vi "dV(dRo).vi"(1 "stop":bool, 4 "dRo /dC":dbl, 6 "dRo %":dbl format="%#_3g", 8 "C подпитка":dbl, 9 "T1к-р C":dbl, 10 "N ГЦП":dbl, 11 "C крайно":dbl) -> (0 "dC г/кг":dbl format="%#_3g", 2 "L см":dbl format="%#_3f", 3 "V м3":dbl format="%#_3f")   [LabVIEW 2023]
panel:
  out "Дозирай на всеки 10 сек за:":dbl format="%#_2g"
  in  "∆L sm":dbl
  in  "F m3/h":dbl
  in  "dN/dt %/h":dbl
  in  "∆N %":dbl
  out "dRo % 2":dbl format="%#_3g"
  in  "dC г/кг 2":dbl format="%#_3g"
  in  "dRo /dC 2":dbl
  out "date/time string":string
  out "V 1к-р":dbl format="%#_3f"
  out "Enum":enum16{"Хов", "Бор"}(ring)
  in  "C начално":dbl
  out "x > y?":bool
  # "сек"
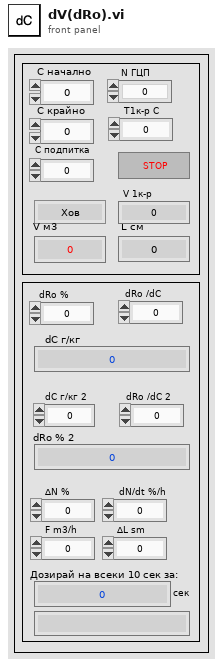
[diagram p1: front panel]
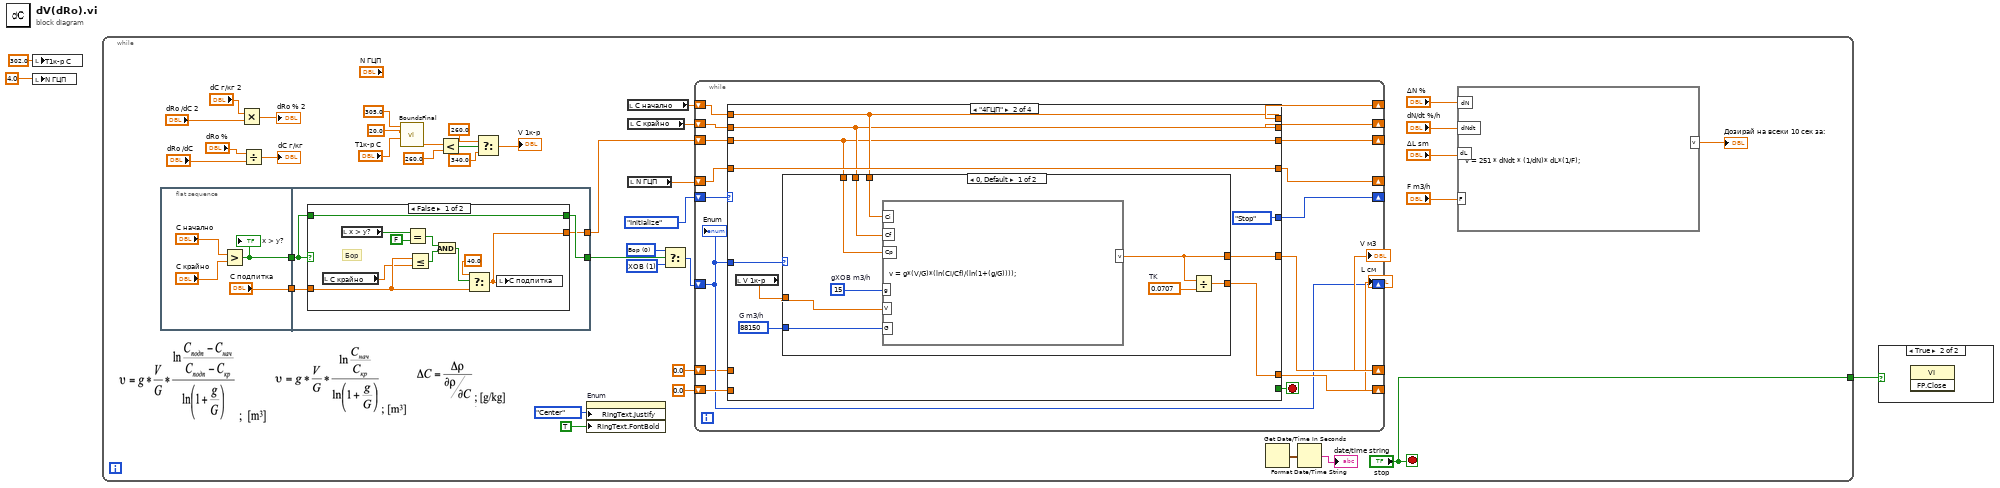
[diagram p0: block diagram]
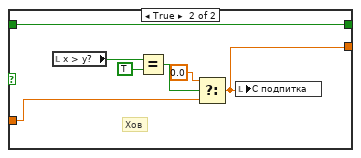
[diagram p3: hidden frame]
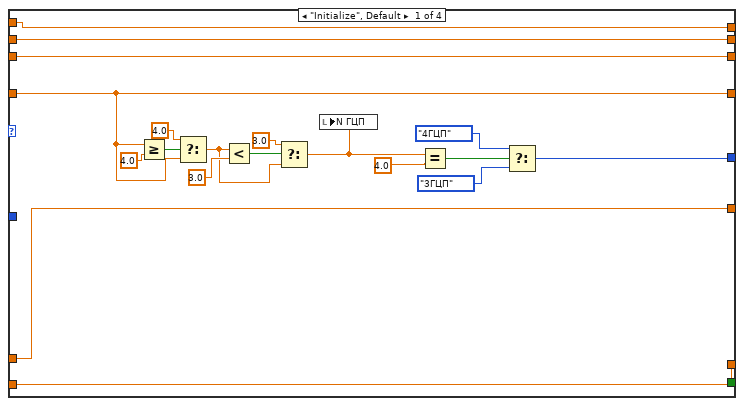
[diagram p4: hidden frame]
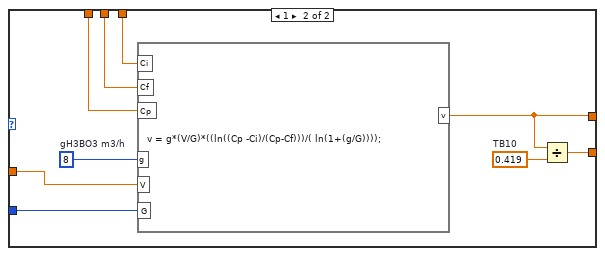
[diagram p5: hidden frame]
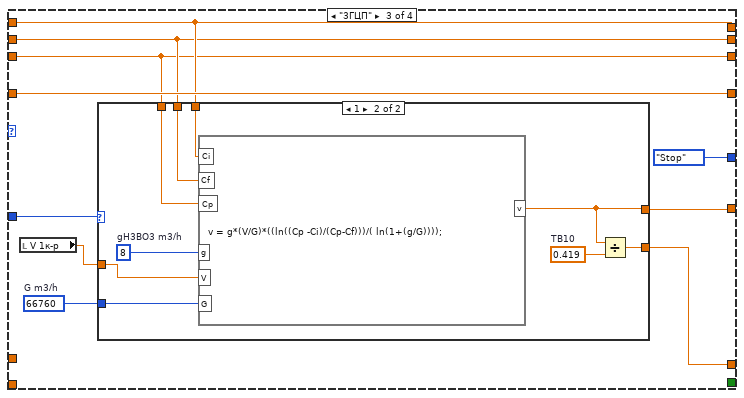
[diagram p6: hidden frame]
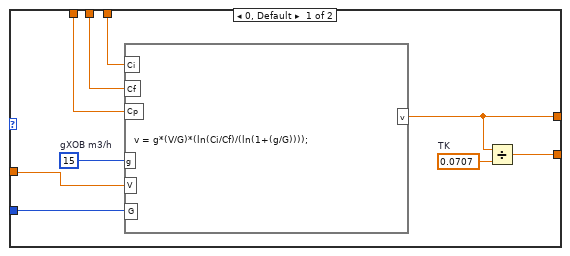
[diagram p7: hidden frame]
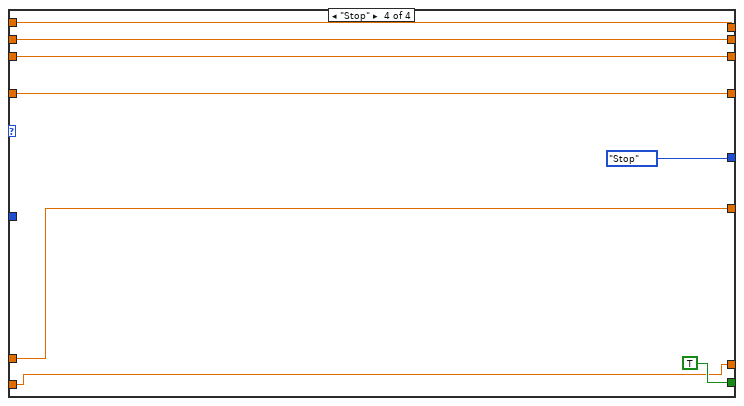
[diagram p8: hidden frame]
diagram:
  n1 = local write "T1к-р C"(302.0) -> ()
  n2 = local write "N ГЦП"(4.0) -> ()
  n3 = while {
    tunnel: ["stop"] -> w3
    stop <- "stop" stop-if-true
    w37 = u16 0 items=["Бор", "ХОВ"]
    w38 = u16 1 items=["Бор", "ХОВ"]
    n4 = flat-sequence {
      tunnel: [w47] -> w43
      tunnel: ["C подпитка"] -> w42
      tunnel: [w50] -> w33
      tunnel: w43 -> [w51]
      tunnel: [w49] -> w32
      tunnel: w42 -> [w48]
      frame #0 {
        n5 = Greater?(x="C начално", y="C крайно") -> (0:w47:bool)
        "x > y?" <- w47
      }
      frame #1 {
        n6 = case shown="False" w51 {
          tunnel: w51 -> [w55 w68]
          tunnel: [w55 w68] -> w50
          tunnel: [w54 w62] -> w49
          tunnel: w48 -> [w53 w63]
          frame False {
            # "Бор"
            n7 = local read "C крайно"() -> (w52:dbl)
            n8 = local read "x > y?"() -> (w58:bool)
            n9 = Equal?(x=w58, y=FALSE) -> (x = y?=w60:bool)
            n10 = Less Or Equal?(x=w53, y=w52) -> (x <= y?=w59:bool)
            n11 = And(x=w60, y=w59) -> (x .and. y?=w61:bool)
            n12 = Select(t=40.0, s=w61, f=w53) -> (s? t:f=w54:dbl)
            n13 = local write "C подпитка"(w54) -> ()
          }
          frame True {
            # "Хов"
            n14 = local read "x > y?"() -> (w66:bool)
            n15 = Equal?(x=w66, y=TRUE) -> (x = y?=w67:bool)
            n16 = Select(t=0.0, s=w67, f=w63) -> (s? t:f=w62:dbl)
            n17 = local write "C подпитка"(w62) -> ()
          }
        }
      }
    }
    n18 = Multiply(x="dC г/кг 2", y="dRo /dC 2") -> (x*y=→"dRo % 2":dbl)
    n19 = Divide(x="dRo %", y="dRo /dC") -> (x/y=→"dC г/кг":dbl)
    n20 = call "BoundsFinal.vi"("N"="T1к-р C", "Low"=20.0, "Hight"=305.0) -> ("Res"=w19:dbl)  [unwired: 8 in]
    n21 = Less?(x=w19, y=260.0) -> (x < y?=w23:bool)
    n22 = Select(t=260.0, s=w23, f=340.0) -> (s? t:f=→"V 1к-р":dbl)
    n23 = property on="Enum" class="Enum (strict)"("RingText.Justify"=enum16{"Left", "Center", "Right"}."Center" ("Ring Text.Justification"), "RingText.FontBold"=TRUE ("Ring Text.Font:Bold")) -> ()  [unwired: 2 in, 2 out]
    n24 = local read "C начално"() -> (w31:dbl)
    n25 = local read "C крайно"() -> (w30:dbl)
    n26 = local read "N ГЦП"() -> (w9:dbl)
    n27 = Select(t=w37, s=w33, f=w38) -> (s? t:f=w39:u16)
    n28 = while {
      shift-right: [w82] -> _
      shift-left: w31 -> [w83]
      shift-right: [w80] -> _
      shift-left: w30 -> [w81]
      shift-right: [w78] -> _
      shift-left: w32 -> [w79]
      shift-right: [w75] -> _
      shift-left: enum16{"Initialize", "4ГЦП", "3ГЦП", "Stop"}."Initialize" -> [w84]
      shift-right: [w76] -> _
      shift-left: w9 -> [w77]
      shift-right: [w72] -> w34
      shift-left: 0.0 ("v") -> [w71]
      shift-right: [w70] -> _
      shift-left: w39 -> [w70]
      shift-right: [w73] -> w36
      shift-left: 0.0 ("v") -> [w69]
      stop <- w74 stop-if-true
      n29 = case shown="\"4ГЦП\"" w84 {
        tunnel: w83 -> [w103 w111 w140 w166]
        tunnel: [w103 w111 w140 w166] -> w82
        tunnel: w81 -> [w102 w110 w139 w165]
        tunnel: [w102 w110 w139 w165] -> w80
        tunnel: w79 -> [w101 w109 w138 w164]
        tunnel: [w101 w109 w138 w164] -> w78
        tunnel: w77 -> [w90 w112 w141 w167]
        tunnel: [w90 w112 w141 w167] -> w76
        tunnel: [w97 enum16{"Initialize", "4ГЦП", "3ГЦП", "Stop"}."Stop" enum16{"Initialize", "4ГЦП", "3ГЦП", "Stop"}."Stop" enum16{"Initialize", "4ГЦП", "3ГЦП", "Stop"}."Stop"] -> w75
        tunnel: [w95 w106 w134 w161] -> w73
        tunnel: [_ _ _ TRUE] -> w74
        tunnel: [w96 w105 w133 w160] -> w72
        tunnel: w71 -> [w96 _ _ w160]
        tunnel: w70 -> [_ w107 w135 _]
        tunnel: w69 -> [w95 _ _ w161]
        frame "Initialize", Default {
          n30 = Greater Or Equal?(x=w90, y=4.0) -> (x >= y?=w92:bool)
          n31 = Select(t=4.0, s=w92, f=w90) -> (s? t:f=w87:dbl)
          n32 = Less?(x=w87, y=3.0) -> (x < y?=w88:bool)
          n33 = Select(t=3.0, s=w88, f=w87) -> (s? t:f=w85:dbl)
          n34 = local write "N ГЦП"(w85) -> ()
          n35 = Equal?(x=w85, y=4.0) -> (x = y?=w100:bool)
          n36 = Select(t=enum16{"Initialize", "4ГЦП", "3ГЦП"}."4ГЦП", s=w100, f=enum16{"Initialize", "4ГЦП", "3ГЦП"}."3ГЦП") -> (s? t:f=w97:enum16{"Initialize", "4ГЦП", "3ГЦП"})
        }
        frame "4ГЦП" {
          w113 = 88150  # G m3/h
          n37 = local read "V 1к-р"() -> (w104:dbl)
          n38 = case shown="0, Default" w107 {
            tunnel: w104 -> [w121 w129]
            tunnel: w113 -> [w122 w130]
            tunnel: w109 -> [w119 w124]
            tunnel: w110 -> [w118 w131]
            tunnel: w111 -> [w117 w123]
            tunnel: [w115 w126] -> w106
            tunnel: [w114 w125] -> w105
            frame 0, Default {
              w116 = 0.0707  # TK
              w120 = 15  # gХОВ m3/h
              n39 = formula code="v = g*(V/G)*(ln(Ci/Cf)/(ln(1+(g/G))));"("Ci"=w117, "Cf"=w118, "Cp"=w119, "g"=w120, "V"=w121, "G"=w122) -> ("v"=w115:dbl)
              n40 = Divide(x=w115, y=w116) -> (x/y=w114:dbl)
            }
            frame 1 {
              w127 = 0.419  # TB10
              w128 = 8  # gH3BO3 m3/h
              n41 = formula code="v = g*(V/G)*((ln((Cp -Ci)/(Cp-Cf)))/( ln(1+(g/G))));"("Ci"=w123, "Cf"=w131, "Cp"=w124, "g"=w128, "V"=w129, "G"=w130) -> ("v"=w126:dbl)
              n42 = Divide(x=w126, y=w127) -> (x/y=w125:dbl)
            }
          }
        }
        frame "3ГЦП" {
          w137 = 66760  # G m3/h
          n43 = local read "V 1к-р"() -> (w132:dbl)
          n44 = case shown="1" w135 {
            tunnel: w132 -> [w149 w155]
            tunnel: w137 -> [w150 w156]
            tunnel: w138 -> [w147 w157]
            tunnel: w139 -> [w146 w158]
            tunnel: w140 -> [w145 w159]
            tunnel: [w143 w151] -> w134
            tunnel: [w142 w152] -> w133
            frame 0, Default {
              w144 = 0.0707  # TK
              w148 = 15  # gХОВ m3/h
              n45 = formula code="v = g*(V/G)*(ln(Ci/Cf)/(ln(1+(g/G))));"("Ci"=w145, "Cf"=w146, "Cp"=w147, "g"=w148, "V"=w149, "G"=w150) -> ("v"=w143:dbl)
              n46 = Divide(x=w143, y=w144) -> (x/y=w142:dbl)
            }
            frame 1 {
              w153 = 0.419  # TB10
              w154 = 8  # gH3BO3 m3/h
              n47 = formula code="v = g*(V/G)*((ln((Cp -Ci)/(Cp-Cf)))/( ln(1+(g/G))));"("Ci"=w159, "Cf"=w158, "Cp"=w157, "g"=w154, "V"=w155, "G"=w156) -> ("v"=w151:dbl)
              n48 = Divide(x=w151, y=w153) -> (x/y=w152:dbl)
            }
          }
        }
        frame "Stop" {
        }
      }
      "Enum" <- w70
    }
    "V м3" <- w36
    "L см" <- w34
    n49 = Get Date/Time In Seconds() -> (seconds since 1Jan1904=w13:timestamp)
    n50 = Format Date/Time String(seconds (now)=w13) -> (date/time string=→"date/time string":string)  [unwired: 2 in]
    n51 = formula code="v = 251 * dNdt * (1/dN)* dL*(1/F);"("dN"="∆N %", "dNdt"="dN/dt %/h", "dL"="∆L sm", "F"="F m3/h") -> ("v"=→"Дозирай на всеки 10 сек за:":dbl)
  }
  n52 = case shown="True" w3 {
    frame False {
    }
    frame True {
      n53 = invoke class="VI" method="FP.Close"() -> ()  [unwired: 3 in, 3 out]
    }
  }
